vi "X_2.91_dashboard.vi"() -> ()   [LabVIEW 2022 SP3]
panel:
  out "data b":dbl
  out "data a":dbl
  in  "load data":bool
  out "randi":dbl
  in  "stop":bool
  out "usr":string
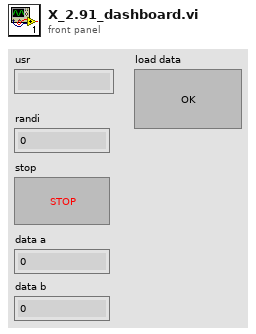
[diagram p1: front panel]
types:
  T1 = enum32{"Invalid", "Standard", "Closed", "Hidden", "Minimized", "Maximized"}
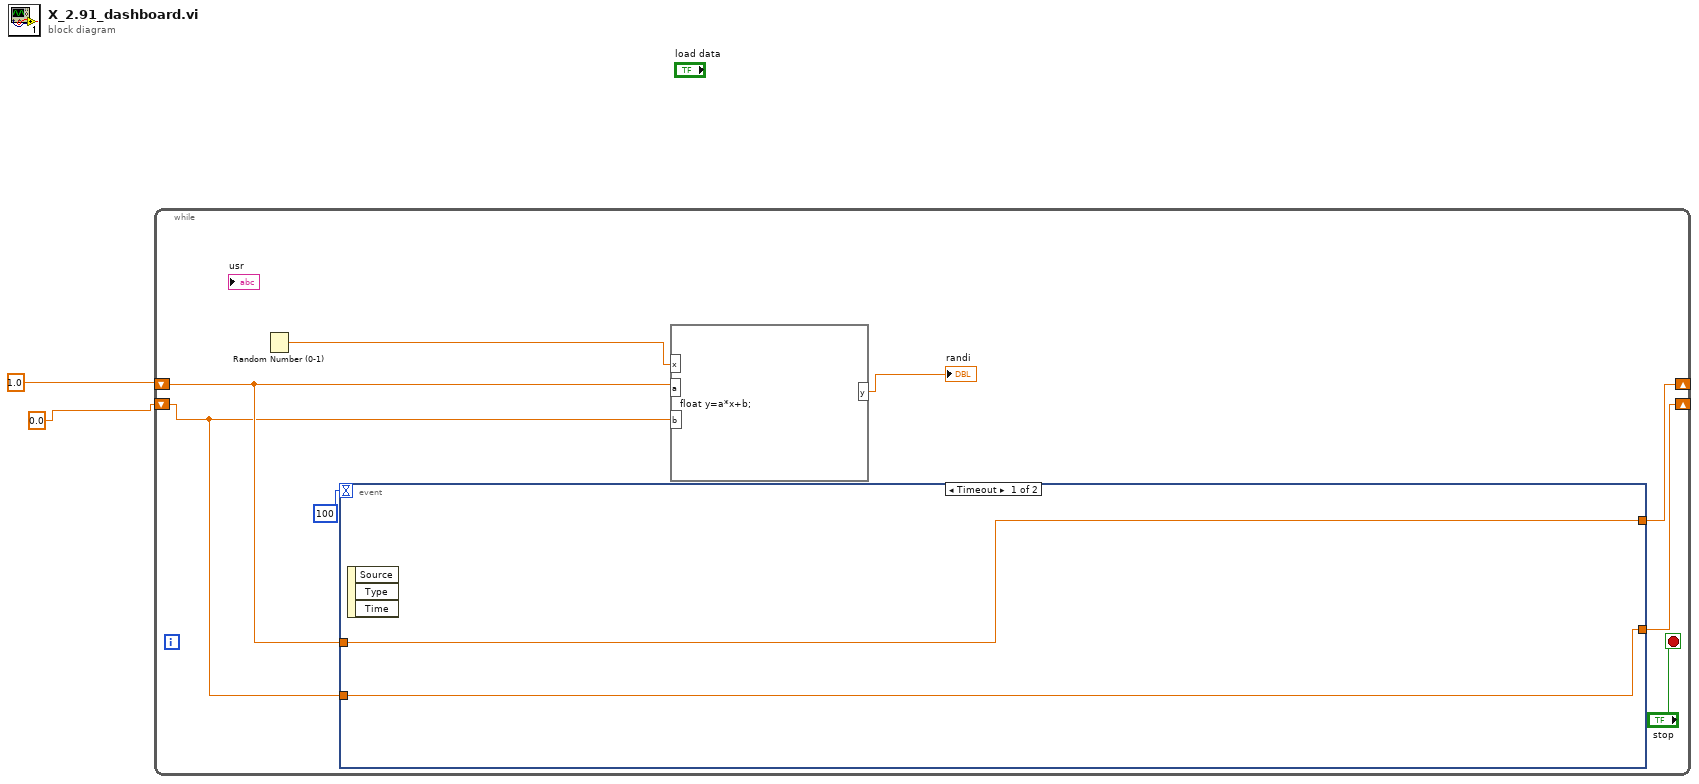
[diagram p0: block diagram]
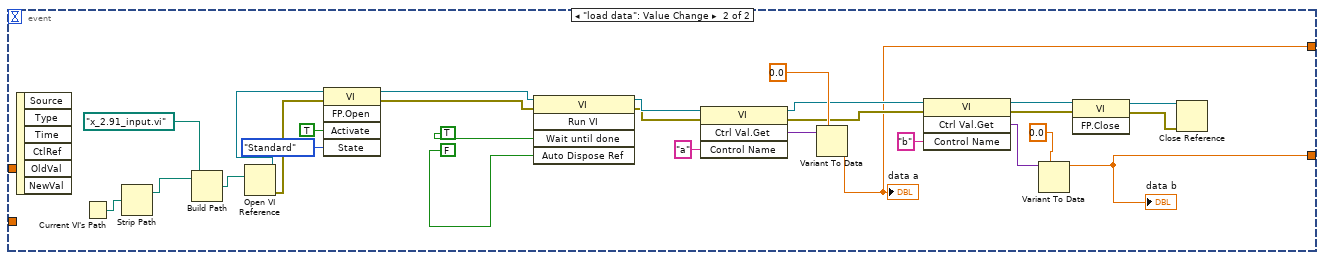
[diagram p2: hidden frame]
diagram:
  n1 = while {
    shift-right: [w5] -> _
    shift-left: 1.0 -> [w4]
    shift-right: [w6] -> _
    shift-left: 0.0 -> [w3]
    stop <- "stop" stop-if-true
    n2 = Random Number (0-1)() -> (number: 0 to 1=w10:dbl)
    n3 = event shown="[0] Timeout" {
      selector: _ -> [_ _]
      dyn-events: _ -> [_ _]
      timeout: 100 -> [_ _]
      tunnel: [w11 w14] -> w6
      tunnel: [w12 w13] -> w5
      tunnel: w4 -> [w12 _]
      tunnel: w3 -> [w11 _]
      event Timeout {
        n4 = event-data() -> ()  [unwired: 1 in, 3 out]
      }
      event "load data": Value Change {
        n5 = event-data() -> ()  [unwired: 1 in, 6 out]
        n6 = Current VI's Path() -> (path=w40:path)
        n7 = Strip Path(path=w40) -> (stripped path=w39:path)  [unwired: 1 out]
        n8 = Build Path(base path=w39, name or relative path=path "x_2.91_input.vi") -> (appended path=w37:path)
        n9 = Open VI Reference(vi path=w37) -> (vi reference=w29:refnum<vi>, error out=w34:errorcluster)  [unwired: 5 in]
        n10 = invoke class="VI" method="FP.Open"(reference=w29, error in=w34, "Activate"=TRUE ("Activate?"), "State"=T1."Standard") -> (reference out=w30:refnum<vi>, error out=w31:errorcluster)  [unwired: 1 in, 3 out]
        n11 = invoke class="VI" method="Run VI"(reference=w30, error in=w31, "Wait until done"=TRUE ("Wait Until Done"), "Auto Dispose Ref"=FALSE ("Auto Dispose Reference")) -> (reference out=w27:refnum<vi>, error out=w26:errorcluster)  [unwired: 1 in, 3 out]
        n12 = invoke class="VI" method="Ctrl Val.Get"(reference=w27, error in=w26, "Control Name"="a") -> (reference out=w21:refnum<vi>, error out=w20:errorcluster, "Get Control Value Variant"=w25:variant)  [unwired: 1 in, 1 out]
        n13 = Variant To Data(type=0.0, Variant=w25) -> (data=w13:dbl)  [unwired: 1 in, 1 out]
        "data a" <- w13
        n14 = invoke class="VI" method="Ctrl Val.Get"(reference=w21, error in=w20, "Control Name"="b") -> (reference out=w19:refnum<vi>, error out=w18:errorcluster, "Get Control Value Variant"=w16:variant)  [unwired: 1 in, 1 out]
        n15 = Variant To Data(type=0.0, Variant=w16) -> (data=w14:dbl)  [unwired: 1 in, 1 out]
        "data b" <- w14
        n16 = invoke class="VI" method="FP.Close"(reference=w19, error in=w18) -> (reference out=w23:refnum<vi>, error out=w22:errorcluster)  [unwired: 1 in, 1 out]
        n17 = Close Reference(reference=w23, error in (no error)=w22) -> ()  [unwired: 1 out]
      }
    }
    n18 = formula code="float y=a*x+b;"("x"=w10, "a"=w4, "b"=w3) -> ("y"=→"randi":dbl)
  }
